vi "Initialize with copy transmission.vi"(8 "error in (no error)":errorcluster, 9 "unit ID":u8=1, 10 "MB copy":refnum<class "Modbus Master CR.lvclass">, 11 "MB in":refnum<class "Modbus Master CR.lvclass">) -> (0 "error out":errorcluster, 3 "MB out":refnum<class "Modbus Master CR.lvclass">)   [LabVIEW 2021, in "Modbus Master CR.lvclass"]
uses:
  Modbus Master CR.lvclass
  Modbus Master CR.lvclass/Modbus Master CR.ctl
  Network Master/Network Master.lvclass
  C:/my_projects/projects/Algorithms/Labview/21/Modbus_v121c/Network Protocol/Network Master/Network Master.lvclass
  C:/my_projects/projects/Algorithms/Labview/21/Modbus_v121c/Network Protocol/Network Protocol.lvclass
  C:/my_projects/projects/Algorithms/Labview/21/Modbus_v121c/Network Protocol/MB/Modbus Master CR.lvclass
  Data Model/Device Data Model.lvclass
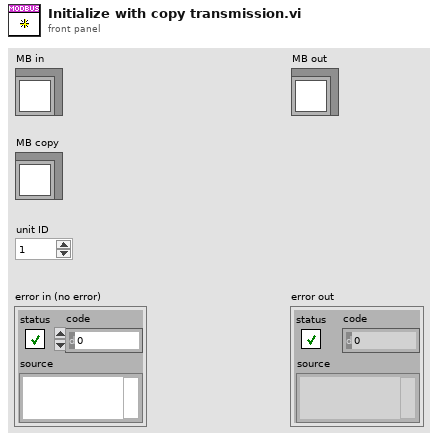
[diagram p1: front panel]
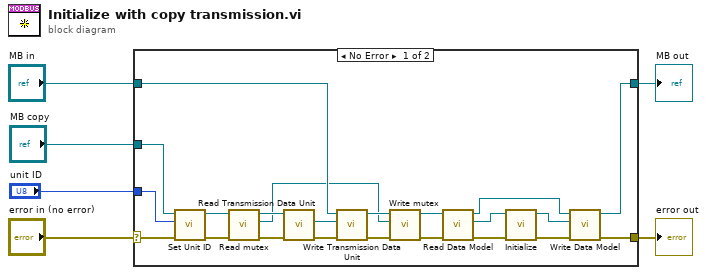
[diagram p0: block diagram]
diagram:
  n1 = case shown="No Error" "error in (no error)" {
    selector: "error in (no error)" -> [w18 w29]
    tunnel: [w22 w29] -> w5
    tunnel: [w23 w30] -> w3
    tunnel: "MB in" -> [w21 w30]
    tunnel: "MB copy" -> [w17 _]
    tunnel: "unit ID" -> [w16 _]
    frame No Error {
      n2 = call "Set Unit ID.vi"("error in (no error)"=w18, "Unit ID"=w16, "Modbus master in"=w17) -> ("error out"=w15:errorcluster, "Modbus master out"=w12:refnum<class "Modbus Master CR.lvclass">)  [unwired: 7 in]
      n3 = call "Read mutex.vi"("error in (no error)"=w15, "Network Master in"=w12) -> ("error out"=w14:errorcluster, "mutex"=w7:refnum<data-value>, "Network Master out"=w13:refnum<class "Modbus Master CR.lvclass">)  [unwired: 7 in]
      n4 = call "Read Transmission Data Unit.vi"("error in (no error)"=w14, "Network Master in"=w13) -> ("error out"=w19:errorcluster, "Transmission Data Unit"=w20:refnum<class "Transmission Data Unit.lvclass">)  [unwired: 7 in, 1 out]
      n5 = call "Write Transmission Data Unit.vi"("error in (no error)"=w19, "Transmission Data Unit"=w20, "Network Master in"=w21) -> ("error out"=w10:errorcluster, "Network Master out"=w11:refnum<class "Modbus Master CR.lvclass">)  [unwired: 7 in]
      n6 = call "Write mutex.vi"("error in (no error)"=w10, "mutex"=w7, "Network Master in"=w11) -> ("error out"=w8:errorcluster, "Network Master in"=w9:refnum<class "Modbus Master CR.lvclass">)  [unwired: 7 in]
      n7 = call "Read Data Model.vi"("error in (no error)"=w8, "MB_TCP in"=w9) -> ("error out"=w27:errorcluster, "Data Model"=w28:refnum<class "Device Data Model.lvclass">, "MB_TCP out"=w24:refnum<class "Modbus Master CR.lvclass">)  [unwired: 7 in]
      n8 = call-dynamic "Initialize.vi"("error in"=w27, "device data model in"=w28) -> ("error out"=w26:errorcluster, "device data model out"=w25:refnum<class "Device Data Model.lvclass">)  [unwired: 8 in]
      n9 = call "Write Data Model.vi"("error in (no error)"=w26, "Data Model"=w25, "MB_TCP in"=w24) -> ("error out"=w22:errorcluster, "MB_TCP out"=w23:refnum<class "Modbus Master CR.lvclass">)  [unwired: 7 in]
    }
    frame Error {
    }
  }
  "error out" <- w5
  "MB out" <- w3
